vi "Kate pop out.vi"(5 "prev iteration":bool, 6 "Window Number (0...15)":i32 min=0 max=15, 7 "pop out":bool, 10 "Title":string, 11 "Image":T1) -> (3 "Image Out (duplicate)":T1)   [LabVIEW 2012]
doc: "SciScan 1.2 160630"
uses:
  <vilib>/vision/Image Controls.llb/IMAQ Image.ctl
panel:
  out "error out":errorcluster
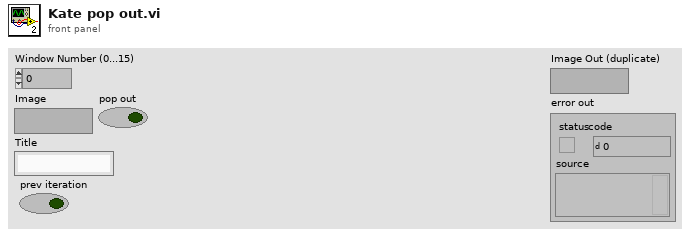
[diagram p1: front panel]
types:
  T1 = typedef "IMAQ Image.ctl" = refnum<image>
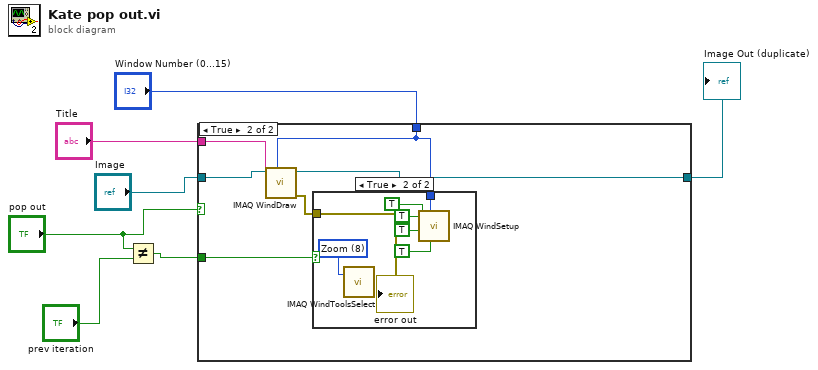
[diagram p0: block diagram]
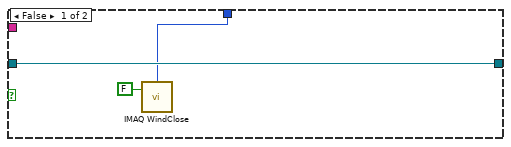
[diagram p2: hidden frame]
diagram:
  n1 = Not Equal?(x="pop out", y="prev iteration") -> (x != y?=w1:bool)
  n2 = case shown="True" "pop out" {
    tunnel: "Window Number (0...15)" -> [w8 w16]
    tunnel: "Image" -> [w9 w15]
    tunnel: [w9 w14] -> w5
    tunnel: "Title" -> [_ w13]
    tunnel: w1 -> [_ w11]
    frame False {
      n3 = call "IMAQ WindClose"("Window Number (0...15)"=w8, "Close All Windows (False)"=FALSE) -> ()  [unwired: 4 in, 1 out]
    }
    frame True {
      n4 = call "IMAQ WindDraw"("Window Number (0...15)"=w16, "Title"=w13, "Image"=w15) -> ("error out"=w12:errorcluster, "Image Out (duplicate)"=w14:T1)  [unwired: 7 in]
      n5 = case shown="True" w11 {
        tunnel: w16 -> [_ w18]
        tunnel: w12 -> [_ w17]
        frame False {
        }
        frame True {
          w19 = u32 8 items=["No Selection", "Point", "Line", "Rectangle", "Oval", "Polygon", "Freehand Region", "Annulus", "Zoom", "Pan", "Broken Line", "Freehand Line", "Rotated Rectangle"] ("Tool (Point)")
          n6 = call "IMAQ WindToolsSelect"("Tool (Point)"=w19) -> ()  [unwired: 4 in, 2 out]
          n7 = call "IMAQ WindSetup"("Window is floating? (No)"=TRUE, "Window Number (0...15)"=w18, "Window has title bar? (Yes)"=TRUE, "Window can close? (Yes)"=TRUE, "Window can grow? (Yes)"=TRUE) -> ()  [unwired: 6 in, 1 out]
          "error out" <- w17
        }
      }
    }
  }
  "Image Out (duplicate)" <- w5
